vi "test_libssh2_session_method_pref.vi"() -> ()   [LabVIEW 2017, in "unit_tests.lvlib"]
uses:
  unit_tests.lvlib
  libssh2/libssh2_method_type.ctl
  libssh2/libssh2_init_default.vi
  libssh2/libssh2_session_init_ex.vi
  libssh2/libssh2.lvlib
  <vilib>/PNR/Transparent Assertions/Transparent Assertions/Transparent Assertions.lvlib
panel:
  out "error out":errorcluster
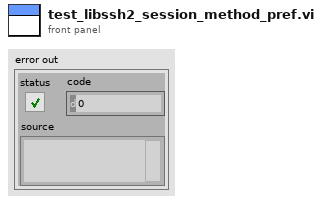
[diagram p1: front panel]
types:
  T1 = typedef "libssh2.lvlib/libssh2_method_type.ctl" = enum16{"LIBSSH2_METHOD_KEX", "LIBSSH2_METHOD_HOSTKEY", "LIBSSH2_METHOD_CRYPT_CS", "LIBSSH2_METHOD_CRYPT_SC", "LIBSSH2_METHOD_MAC_CS", "LIBSSH2_METHOD_MAC_SC", "LIBSSH2_METHOD_COMP_CS", "LIBSSH2_METHOD_COMP_SC", "LIBSSH2_METHOD_LANG_CS", "LIBSSH2_METHOD_LANG_SC", "LIBSSH2_METHOD_SIGN_ALGO"}
  T2 = typedef "libssh2.lvlib/Session Refnum.ctl" = refnum<k1>
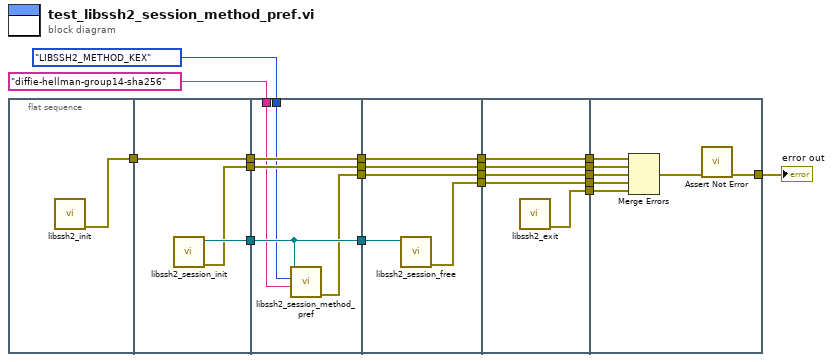
[diagram p0: block diagram]
diagram:
  n1 = flat-sequence {
    tunnel: [w21] -> w4
    tunnel: w4 -> [w24]
    tunnel: [w24] -> w16
    tunnel: [w23] -> w15
    tunnel: [w22] -> w14
    tunnel: w16 -> [w30]
    tunnel: [w30] -> w10
    tunnel: w15 -> [w28]
    tunnel: [w28] -> w9
    tunnel: w14 -> [w29]
    tunnel: [w29] -> w8
    tunnel: libssh2_method_type."LIBSSH2_METHOD_KEX" ("method_type") -> [w27]
    tunnel: "diffie-hellman-group14-sha256" -> [w26]
    tunnel: [w25] -> w3
    tunnel: w10 -> [w35]
    tunnel: [w35] -> w7
    tunnel: w9 -> [w34]
    tunnel: w8 -> [w33]
    tunnel: [w33] -> w6
    tunnel: [w32] -> w5
    tunnel: w3 -> [w31]
    tunnel: [w31] -> w2
    tunnel: w7 -> [w40]
    tunnel: [w40] -> w20
    tunnel: [w39] -> w19
    tunnel: w6 -> [w38]
    tunnel: [w38] -> w18
    tunnel: w5 -> [w37]
    tunnel: [w37] -> w17
    tunnel: w2 -> [w36]
    tunnel: [w36] -> w1
    tunnel: w20 -> [w47]
    tunnel: w19 -> [w46]
    tunnel: w18 -> [w45]
    tunnel: w17 -> [w44]
    tunnel: [w42] -> w11
    tunnel: w1 -> [w41]
    frame #0 {
      n2 = call-poly "libssh2_init.vi"() -> ("error out"=w21:errorcluster)  [unwired: 11 in]
    }
    frame #1 {
      n3 = call "libssh2_session_init.vi"() -> ("error out"=w22:errorcluster, "session"=w23:T2)  [unwired: 10 in]
    }
    frame #2 {
      n4 = call "libssh2_session_method_pref.vi"("prefs"=w26, "method_type"=w27, "session"=w28) -> ("error out"=w25:errorcluster)  [unwired: 8 in]
    }
    frame #3 {
      n5 = call "libssh2_session_free.vi"("session"=w34) -> ("error out"=w32:errorcluster)  [unwired: 10 in]
    }
    frame #4 {
      n6 = call "libssh2_exit.vi"() -> ("error out"=w39:errorcluster)  [unwired: 11 in]
    }
    frame #5 {
      n7 = Merge Errors(w47, w45, w41, w44, w46) -> (w43:errorcluster)
      n8 = call <vilib>:"Assert Not Error.vi"("error in (no error)"=w43) -> ("error out"=w42:errorcluster)  [unwired: 10 in]
    }
  }
  "error out" <- w11
